vi "ROS_Loop_Rate.vi"(3 "Loop Rate (Hz)":dbl, 6 "error in":errorcluster) -> (0 "Time Waited":i32, 5 "error out":errorcluster)   [LabVIEW 2012]
doc: "Attempts to force the loop containing this vi to run at a constant rate. If the desired loop rate is faster than the loop is executing, this will do nothing."
panel:
  out "msec/loop":dbl
  out "Time in Loop":u32
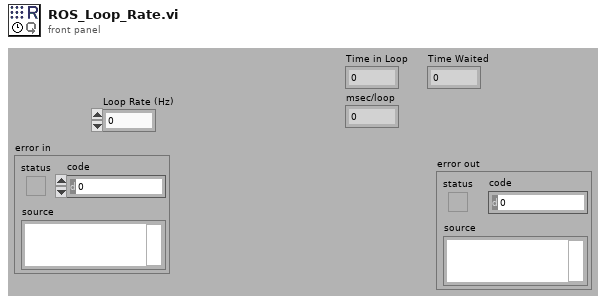
[diagram p1: front panel]
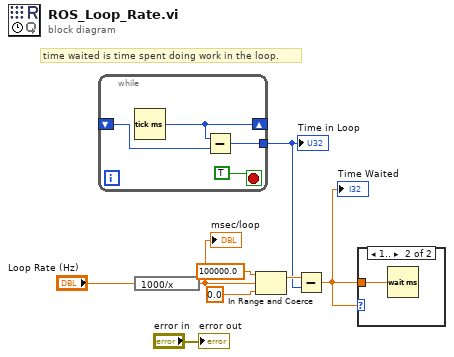
[diagram p0: block diagram]
diagram:
  # "time waited is time spent doing work in the loop."
  n1 = while {
    shift-right: [w12] -> _
    shift-left: _ -> [w11]
    tunnel: [w9] -> w4
    stop <- TRUE stop-if-true
    n2 = Tick Count (ms)() -> (millisecond timer value=w12:u32)
    n3 = Subtract(x=w12, y=w11) -> (x-y=w9:u32)
  }
  "Time in Loop" <- w4
  n4 = expression code="1000/x"("Loop Rate (Hz)") -> (w8:dbl)
  "msec/loop" <- w8
  n5 = In Range and Coerce(upper limit=100000.0, x=w8, lower limit=0.0) -> (coerced(x)=w5:dbl)  [unwired: 1 out]
  n6 = Subtract(x=w5, y=w4) -> (x-y=w2:dbl)
  "Time Waited" <- w2
  n7 = case shown="1.." w2 {
    tunnel: w2 -> [_ w13]
    frame Default {
    }
    frame 1.. {
      n8 = Wait (ms)(milliseconds to wait=w13) -> ()  [unwired: 1 out]
    }
  }
  "error out" <- "error in"
